vi "FlushOneMessageFromQue.vi"(6 "Mode":bool, 8 "error in (no error)":errorcluster, 9 "MsgToRemove":string, 11 "Message que":T1) -> (0 "error out":errorcluster, 3 "Message que out":T1)   [LabVIEW 2017]
doc: "remove all commands/messages of a single name from the que."
uses:
  MessageQue.ctl
  MessageCluster.ctl
  MessageQue.lvlib
panel:
  out "removed messages":i16
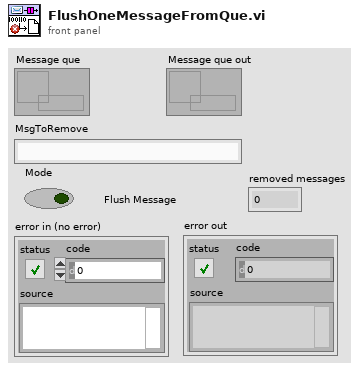
[diagram p1: front panel]
types:
  T1 = typedef "MessageQue.lvlib/MessageQue.ctl" = refnum<queue>
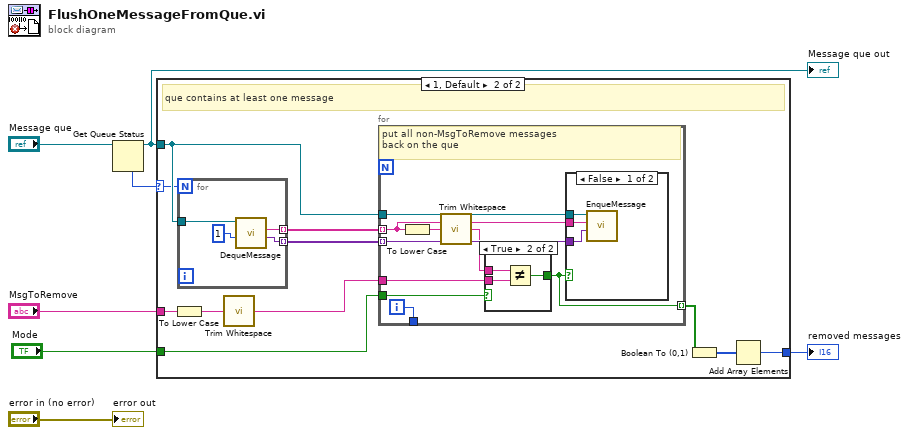
[diagram p0: block diagram]
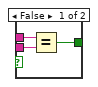
[diagram p3: hidden frame]
diagram:
  n1 = Get Queue Status(queue="Message que") -> (queue out=w4:T1, # elements in queue=w3:i32)  [unwired: 2 in, 6 out]
  "Message que out" <- w4
  n2 = case shown="1, Default" w3 {
    selector: w3 -> [_ w15]
    tunnel: "MsgToRemove" -> [_ w18]
    tunnel: w4 -> [_ w17]
    tunnel: [_ w9] -> w2
    tunnel: "Mode" -> [_ w8]
    frame 0 {
      # "empty que"
    }
    frame 1, Default {
      # "que contains at least one message"
      n3 = To Lower Case(string=w18) -> (all lower case string=w13:string)
      n4 = for {
        N: w15 -> [_]
        tunnel: w17 -> [w39]
        tunnel: [w38] -> w14 mode=indexing
        tunnel: [w37] -> w16 mode=indexing
        n5 = call "DequeMessage.vi"("timeout in ms (-1)"=1, "Message que"=w39) -> ("Message Payload"=w37:variant, "Message Command"=w38:string)  [unwired: 4 in, 4 out]
      }
      n6 = call <vilib>:"Trim Whitespace.vi"("string"=w13) -> ("trimmed string"=w12:string)  [unwired: 1 in]
      n7 = for {
        tunnel: w17 -> [w27]
        tunnel: w14 -> [w24] mode=indexing
        tunnel: w16 -> [w26] mode=indexing
        tunnel: w12 -> [w22]
        tunnel: [w21] -> _
        tunnel: [w20] -> w11 mode=indexing
        tunnel: w8 -> [w19]
        i -> [w21]
        # "put all non-MsgToRemove messages \nback on the que"
        n8 = To Lower Case(string=w24) -> (all lower case string=w25:string)
        n9 = call <vilib>:"Trim Whitespace.vi"("string"=w25) -> ("trimmed string"=w23:string)  [unwired: 1 in]
        n10 = case shown="True" w19 {
          tunnel: w23 -> [w30 w32]
          tunnel: w22 -> [w29 w31]
          tunnel: [w28 w33] -> w20
          frame False {
            n11 = Equal?(x=w30, y=w29) -> (x = y?=w28:bool)
          }
          frame True {
            n12 = Not Equal?(x=w32, y=w31) -> (x != y?=w33:bool)
          }
        }
        n13 = case shown="False" w20 {
          tunnel: w27 -> [w36 _]
          tunnel: w24 -> [w35 _]
          tunnel: w26 -> [w34 _]
          frame False {
            n14 = call "EnqueMessage.vi"("Message Payload"=w34, "Message Command"=w35, "Message que"=w36) -> ()  [unwired: 7 in, 2 out]
          }
          frame True {
            # "remove this msg"
          }
        }
      }
      n15 = Boolean To (0,1)(Boolean=w11) -> (0, 1=w10:i16[])
      n16 = Add Array Elements(numeric array=w10) -> (sum=w9:i16)
    }
  }
  "removed messages" <- w2
  "error out" <- "error in (no error)"
